vi "PD Detection Display 4.vi"() -> ()   [LabVIEW 2014]
uses:
  <vilib>/Instr/_visa.llb/VISA Open Access Mode.ctl
  <vilib>/Instr/_visa.llb/VISA Flush IO Buffer Mask.ctl
  <vilib>/Instr/_visa.llb/VISA Configure Serial Port (Instr).vi
  <vilib>/Utility/file.llb/Write To Spreadsheet File (DBL).vi
panel:
  in  "VISA resource name":refnum<visa-resource-name>="COM4"
  in  "Notes":string="data"
  in  "Save Histogram?":bool=TRUE
  in  "Num Samples":u64=10000
  in  "Samples":bool
  out "PD/s (now)":dbl
  out "Bytes at Port":u32
  out "PD/s (total)":dbl
  out "raw data":string
  out "Waveform Chart":dbl[](graph)
  out "array":dbl[](array[numeric])
  out "Packets at Port":u32
  in  "stop":bool
  # "Infinite"
  # "This Many ->"
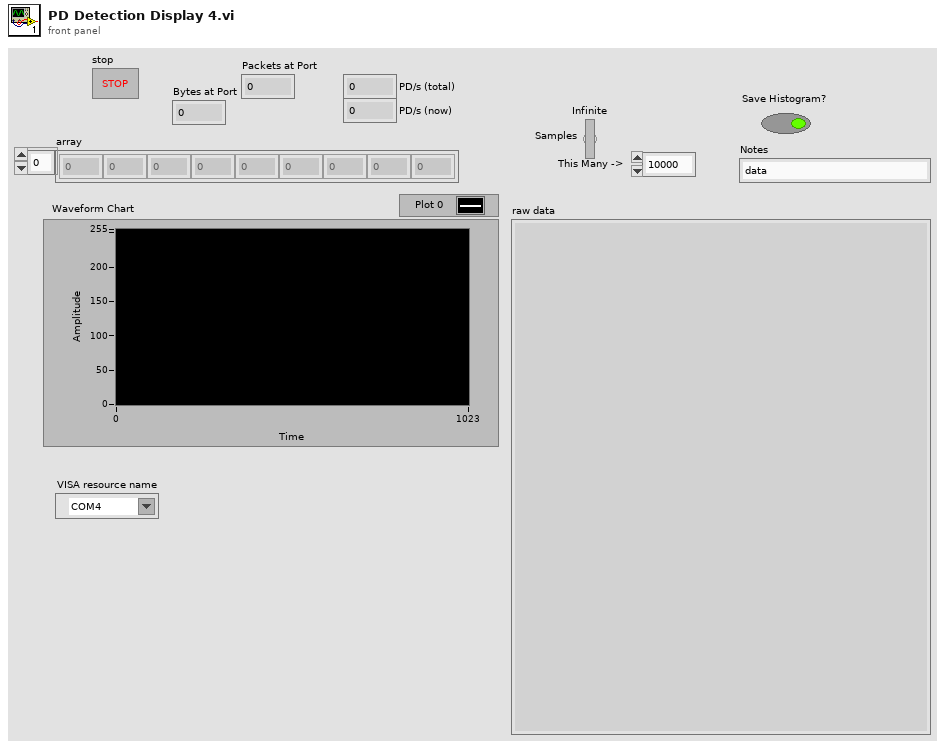
[diagram p1: front panel]
types:
  T1 = typedef "VISA Flush IO Buffer Mask.ctl" = u16
  T2 = typedef "VISA Open Access Mode.ctl" = u32
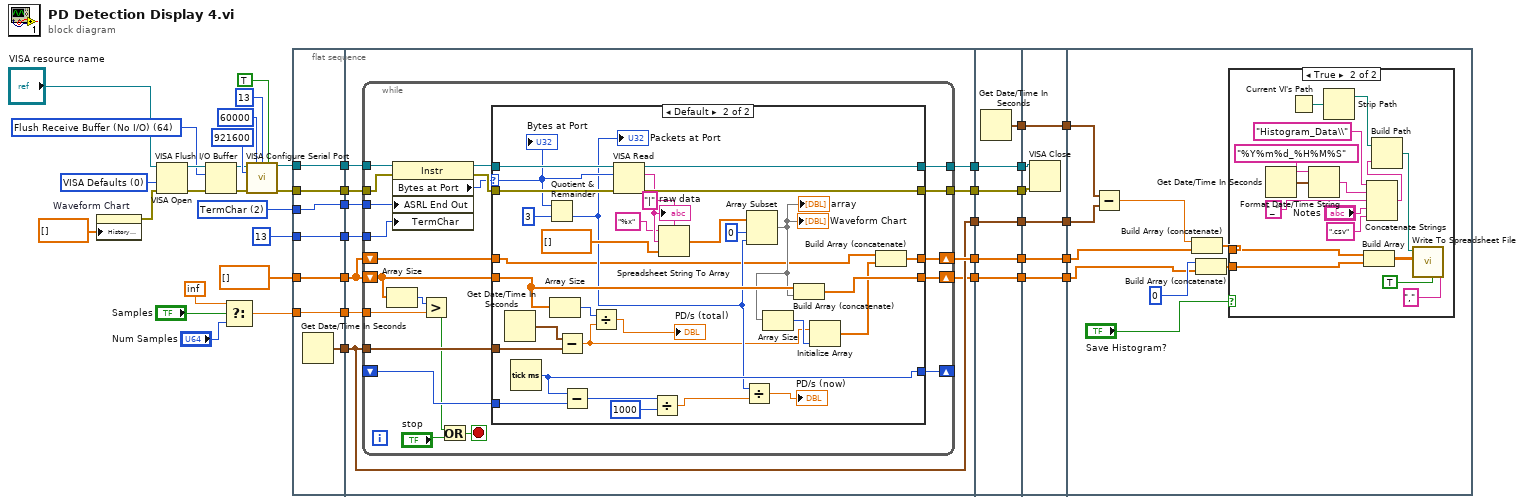
[diagram p0: block diagram]
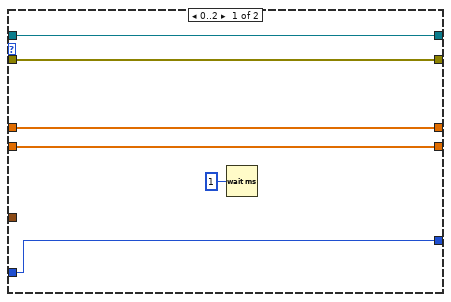
[diagram p2: hidden frame]
diagram:
  w12 = u16 2 items=["None", "Last Bit", "TermChar", "Break"] ("Serial Settings:End Mode for Writes")
  w34 = T1 64 items=["Flush Receive Buffer"=16, "Write Transmit Buffer to Device"=32, "Flush Receive Buffer (No I/O)"=64, "Flush Transmit Buffer"=128] ("Mask")
  w41 = T2 0 items=["VISA Defaults"=0, "Exclusive Lock"=1, "Load Configured Settings"=4] ("Access Mode")
  n1 = property on="Waveform Chart" class="WFChart (strict)"("History Data"=dbl[] []) -> (error out=w33:errorcluster)  [unwired: 2 in, 1 out]
  n2 = VISA Open(access mode=w41, error in (no error)=w33, VISA resource name="VISA resource name") -> (VISA resource name=w37:refnum<visa-resource-name>, error out=w38:errorcluster)  [unwired: 2 in]
  n3 = VISA Flush I/O Buffer(VISA resource name=w37, mask (16)=w34, error in (no error)=w38) -> (VISA resource name out=w35:refnum<visa-resource-name>, error out=w36:errorcluster)
  n4 = Select(t=inf, s="Samples", f="Num Samples") -> (s? t:f=w5:dbl)
  n5 = call-poly "VISA Configure Serial Port"("VISA resource name"=w35, "timeout (10sec)"=u32 60000, "termination char\n(0xA = '\\n' = LF)"=u8 13 ("termination char\n(0xA = '\\n' = LF)"), "Enable Termination\nChar (T)"=TRUE ("Enable Termination\nChar (T)"), "baud rate (9600)"=u32 921600, "error in (no error)"=w36) -> ("VISA resource name out"=w15:refnum<visa-resource-name>, "error out"=w14:errorcluster)  [unwired: 8 in]
  n6 = flat-sequence {
    tunnel: [w51] -> w17
    tunnel: [w50] -> w16
    tunnel: w15 -> [w50]
    tunnel: w14 -> [w49]
    tunnel: [w49] -> w13
    tunnel: w12 -> [w48]
    tunnel: [w48] -> w11
    tunnel: u8 13 ("termination char\n(0xA = '\\n' = LF)") -> [w47]
    tunnel: [w47] -> w9
    tunnel: dbl[] [] -> [w46]
    tunnel: [w46] -> w7
    tunnel: [w45] -> w6
    tunnel: w5 -> [w45]
    tunnel: [w60] -> w20
    tunnel: [w62] -> w19
    tunnel: [w61] -> w18
    tunnel: w17 -> [w54]
    tunnel: w16 -> [w59]
    tunnel: w13 -> [w58]
    tunnel: w11 -> [w57]
    tunnel: w9 -> [w56]
    tunnel: w7 -> [w53]
    tunnel: w6 -> [w55]
    tunnel: [w54] -> w4
    tunnel: [w52] -> w1
    tunnel: [w126] -> w26
    tunnel: [w125] -> w25
    tunnel: [w124] -> w23
    tunnel: [w123] -> w22
    tunnel: [w122] -> w21
    tunnel: w20 -> [w126]
    tunnel: w19 -> [w123]
    tunnel: w18 -> [w122]
    tunnel: w4 -> [w125]
    tunnel: [w121] -> w2
    tunnel: w1 -> [w121]
    tunnel: [w132] -> w28
    tunnel: [w131] -> w27
    tunnel: w26 -> [w132]
    tunnel: w25 -> [w131]
    tunnel: [w130] -> w24
    tunnel: w23 -> [w130]
    tunnel: w22 -> [w129]
    tunnel: w21 -> [w128]
    tunnel: [w127] -> w3
    tunnel: w2 -> [w127]
    tunnel: w28 -> [w133]
    tunnel: w27 -> [w140]
    tunnel: w24 -> [w135]
    tunnel: w3 -> [w134]
    frame #0 {
      n7 = Get Date/Time In Seconds() -> (seconds since 1Jan1904=w51:timestamp)
    }
    frame #1 {
      n8 = while {
        tunnel: [w83] -> w61
        tunnel: [w82] -> w62
        tunnel: w59 -> [w78]
        tunnel: w58 -> [w79]
        shift-right: [w81] -> w52
        shift-left: w53 -> [w70]
        tunnel: w54 -> [w80]
        tunnel: w57 -> [w74]
        tunnel: w56 -> [w73]
        shift-right: [w72] -> _
        shift-left: _ -> [w71]
        tunnel: w55 -> [w69]
        shift-right: [w64] -> w60
        shift-left: w53 -> [w63]
        stop <- w67 stop-if-true
        n9 = Array Size(array=w70) -> (size(s)=w68:i32)
        n10 = property class="Instr"(reference=w78, error in=w79, "ASRL End Out"=w74, "TermChar"=w73) -> (reference out=w77:refnum<visa-resource-name>, error out=w76:errorcluster, "Bytes at Port"=w75:u32)
        n11 = Greater?(x=w68, y=w69) -> (0:w66:bool)
        n12 = Or(x=w66, y="stop") -> (x .or. y?=w67:bool)
        n13 = case shown="Default" w75 {
          selector: w75 -> [_ w101]
          tunnel: [w88 w119] -> w83
          tunnel: [w89 w118] -> w82
          tunnel: w76 -> [w88 w120]
          tunnel: w77 -> [w89 w117]
          tunnel: [w87 w113] -> w81
          tunnel: w70 -> [w87 w112]
          tunnel: w80 -> [_ w110]
          tunnel: [w85 w105] -> w72
          tunnel: w71 -> [w85 w107]
          tunnel: [w84 w91] -> w64
          tunnel: w63 -> [w84 w92]
          frame 0..2 {
            n14 = Wait (ms)(milliseconds to wait=u32 1) -> ()  [unwired: 1 out]
          }
          frame Default {
            n15 = Get Date/Time In Seconds() -> (seconds since 1Jan1904=w108:timestamp)
            n16 = Tick Count (ms)() -> (millisecond timer value=w105:u32)
            n17 = Quotient & Remainder(x=w101, y=u32 3) -> (floor(x/y)=w98:u32)  [unwired: 1 out]
            "Packets at Port" <- w98
            n18 = Array Size(array=w112) -> (size(s)=w111:i32)
            n19 = Subtract(x=w108, y=w110) -> (x-y=w94:dbl)
            n20 = Subtract(x=w105, y=w107) -> (x-y=w104:u32)
            n21 = Divide(x=w111, y=w94) -> (x/y=→"PD/s (total)":dbl)
            n22 = VISA Read(VISA resource name=w117, byte count=w101, error in (no error)=w120) -> (VISA resource name out=w118:refnum<visa-resource-name>, read buffer=w115:string, error out=w119:errorcluster)  [unwired: 1 out]
            "raw data" <- w115
            n23 = Divide(x=w104, y=u32 1000) -> (x/y=w103:dbl)
            n24 = Spreadsheet String To Array(delimiter (Tab)="|", format string="%x", spreadsheet string=w115, array type (2D Dbl)=dbl[] []) -> (array=w99:dbl[])
            n25 = Divide(x=w98, y=w103) -> (x/y=→"PD/s (now)":dbl)
            n26 = Array Subset(array=w99, index=0, length=w98) -> (w96:dbl[])
            "array" <- w96
            "Waveform Chart" <- w96
            n27 = Array Size(array=w96) -> (size(s)=w95:i32)
            n28 = Build Array (concatenate)(w112, w96) -> (w113:dbl[])
            n29 = Initialize Array(w94, w95) -> (w93:dbl[])
            n30 = Build Array (concatenate)(w92, w93) -> (w91:dbl[])
            "Bytes at Port" <- w101
          }
        }
      }
    }
    frame #2 {
      n31 = Get Date/Time In Seconds() -> (seconds since 1Jan1904=w124:timestamp)
    }
    frame #3 {
      n32 = VISA Close(VISA resource name=w129, error in (no error)=w128) -> ()  [unwired: 1 out]
    }
    frame #4 {
      n33 = Subtract(x=w135, y=w140) -> (x-y=w138:dbl)
      n34 = Build Array (concatenate)(w138, w133) -> (w137:dbl[])
      n35 = Build Array (concatenate)(0, w134) -> (w139:dbl[])
      n36 = case shown="True" "Save Histogram?" {
        tunnel: w137 -> [_ w143]
        tunnel: w139 -> [_ w142]
        frame False {
        }
        frame True {
          n37 = Get Date/Time In Seconds() -> (seconds since 1Jan1904=w156:timestamp)
          n38 = Current VI's Path() -> (path=w152:path)
          n39 = Format Date/Time String(time format string (%c)="%Y%m%d_%H%M%S", seconds (now)=w156) -> (date/time string=w153:string)  [unwired: 1 in]
          n40 = Strip Path(path=w152) -> (stripped path=w151:path)  [unwired: 1 out]
          n41 = Build Array(w143, w142) -> (w157:dbl[][])
          n42 = Concatenate Strings("Histogram_Data\\", w153, "_", "Notes", ".csv") -> (w150:string)
          n43 = Build Path(base path=w151, name or relative path=w150) -> (appended path=w149:path)
          n44 = call-poly <vilib>:"Write To Spreadsheet File.vi"("delimiter (\\t)"="," ("delimiter (\\t)"), "transpose? (no:F)"=TRUE, "2D data"=w157, "file path (dialog if empty)"=w149) -> ()  [unwired: 4 in, 1 out]
        }
      }
    }
  }
